vi "Asterisk_header.vi"(1 "Channel names":string[](array[string])) -> (0 "Header string":string)   [LabVIEW 2010]
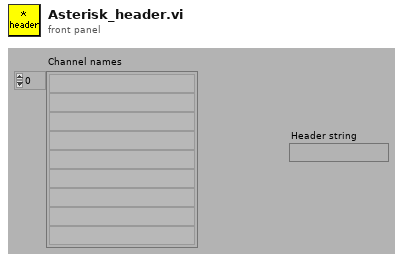
[diagram p1: front panel]
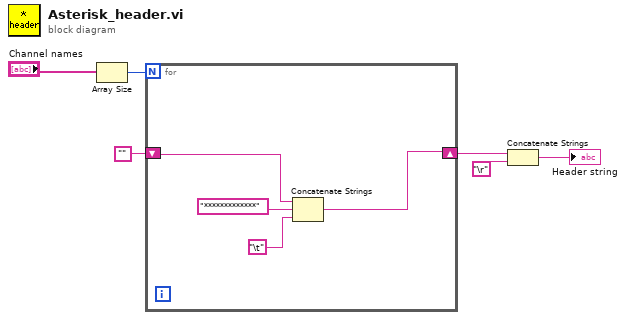
[diagram p0: block diagram]
diagram:
  n1 = Array Size(array="Channel names") -> (size(s)=w2:i32)
  n2 = for {
    N: w2 -> [_]
    shift-right: [w7] -> w4
    shift-left: "" -> [w8]
    n3 = Concatenate Strings(w8, "*************", "\t") -> (w7:string)
  }
  n4 = Concatenate Strings(w4, "\r") -> (→"Header string":string)
